vi "Write Data to Buffer.vi"(8 "error in (no error)":errorcluster, 10 "Data":variant, 11 "Hardware in":refnum<class "Hardware.lvclass">) -> (0 "error out":errorcluster, 3 "Hardware out":refnum<class "Hardware.lvclass">)   [LabVIEW 2017, in "Hardware.lvlib" / "Hardware.lvclass"]
uses:
  Hardware.lvclass
  Hardware.lvclass/Hardware.ctl
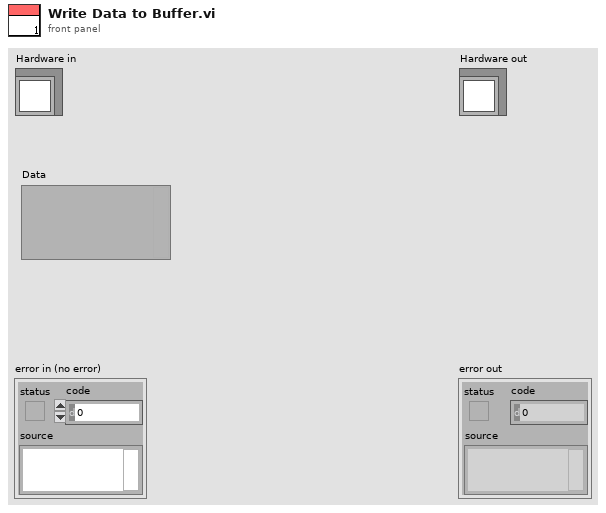
[diagram p1: front panel]
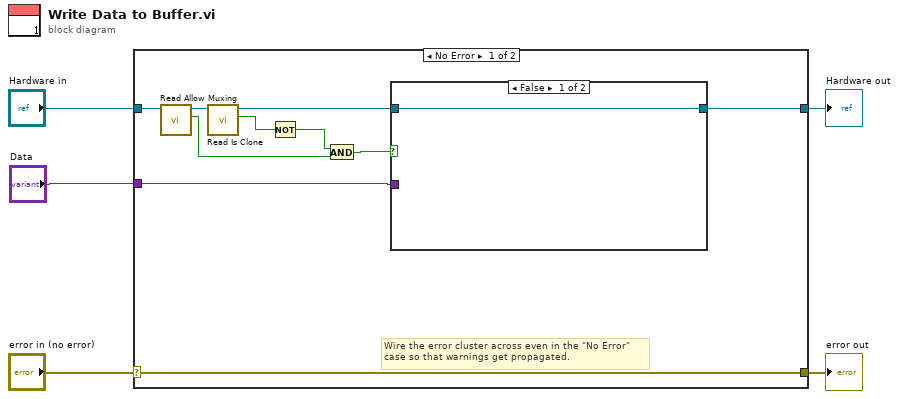
[diagram p0: block diagram]
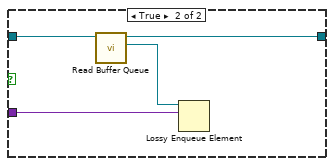
[diagram p2: hidden frame]
diagram:
  n1 = case shown="No Error" "error in (no error)" {
    selector: "error in (no error)" -> [w15 w22]
    tunnel: [w15 w22] -> w4
    tunnel: [w14 w21] -> w2
    tunnel: "Hardware in" -> [w11 w21]
    tunnel: "Data" -> [w13 _]
    frame No Error {
      # "Wire the error cluster across even in the \"No Error\"\ncase so that warnings get propagated."
      n2 = call "Read Allow Muxing.vi"("Hardware in"=w11) -> ("Allow Muxing"=w9:bool, "Hardware out"=w10:refnum<class "Hardware.lvclass">)  [unwired: 8 in, 1 out]
      n3 = call "Read Is Clone.vi"("Hardware in"=w10) -> ("Is Clone?"=w8:bool, "Hardware out"=w12:refnum<class "Hardware.lvclass">)  [unwired: 8 in, 1 out]
      n4 = Not(x=w8) -> (.not. x?=w7:bool)
      n5 = And(x=w7, y=w9) -> (x .and. y?=w6:bool)
      n6 = case shown="False" w6 {
        tunnel: [w16 w20] -> w14
        tunnel: w13 -> [_ w18]
        tunnel: w12 -> [w16 w17]
        frame False {
        }
        frame True {
          n7 = call "Read Buffer Queue.vi"("Hardware in"=w17) -> ("Buffer Queue"=w19:refnum<queue>, "Hardware out"=w20:refnum<class "Hardware.lvclass">)  [unwired: 8 in, 1 out]
          n8 = Lossy Enqueue Element(queue=w19, element=w18) -> ()  [unwired: 1 in, 4 out]
        }
      }
    }
    frame Error {
    }
  }
  "error out" <- w4
  "Hardware out" <- w2
